vi "Switch Scalar Type.vi"(8 "error in (no error)":errorcluster, 11 "Node Ptr":u64 format="%.0x") -> (0 "error out":errorcluster)   [LabVIEW 2020, in "FPGA Addon System Explorer.lvlib"]
uses:
  FPGA Addon System Explorer.lvlib
  <vilib>/NI VeriStand/Custom Device Tools/Custom Device Utility Library/Search Direction.ctl
  <vilib>/NI VeriStand/Custom Device API/Custom Device Channel.ctl
  <vilib>/NI VeriStand/Custom Device API/Custom Device Channel Type.ctl
  Addon Shared/SubVIs/Constants.vi
  <vilib>/NI VeriStand/Custom Device Tools/Custom Device Utility Library/NI VeriStand - Search for Item by GUID.vi
  <vilib>/NI VeriStand/Custom Device API/Get Item Property (String).vi
  <vilib>/NI VeriStand/Custom Device API/Set Item Property (String).vi
  <vilib>/NI VeriStand/Custom Device API/Custom Device API.lvlib
  Addon Shared/FPGA Addon Shared.lvlib
  <vilib>/NI VeriStand/Custom Device Tools/Custom Device Utility Library/Custom Device Utility Library.lvlib
panel:
  in  "Tag":string
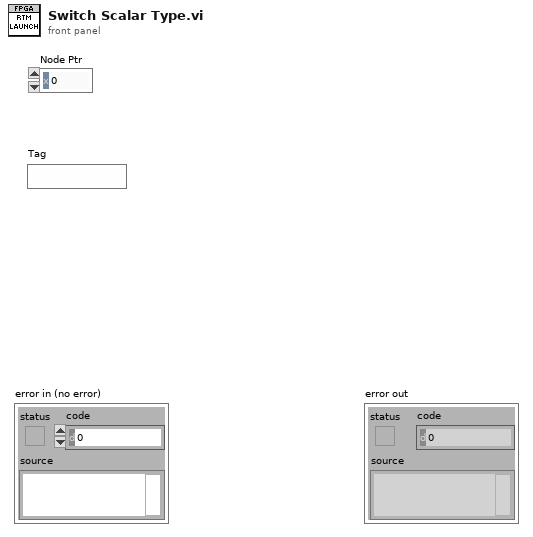
[diagram p1: front panel]
types:
  T1 = typedef "Custom Device Utility Library.lvlib/Search Direction.ctl" = enum16{"Down", "Up"}
  T2 = typedef "Custom Device API.lvlib/Custom Device Item Ref.ctl" = u64
  T3 = typedef "Custom Device API.lvlib/Custom Device Item Info.ctl" = cluster{"Name":string, "Is Channel":bool, "GUID":string, "Is Waveform":bool}
  T4 = typedef "Custom Device API.lvlib/Custom Device Channel.ctl" = cluster{"Type":T5, "Units":string, "Default Value":dbl, "Faultable":bool, "Scalable":bool}
  T5 = typedef "Custom Device API.lvlib/Custom Device Channel Type.ctl" = enum16{"Input", "Output"}
  T6 = enum32{"invalid app kind", "Development System", "Run Time System", "Student Edition", "Embedded LabVIEW", "Evaluation", "Custom"}
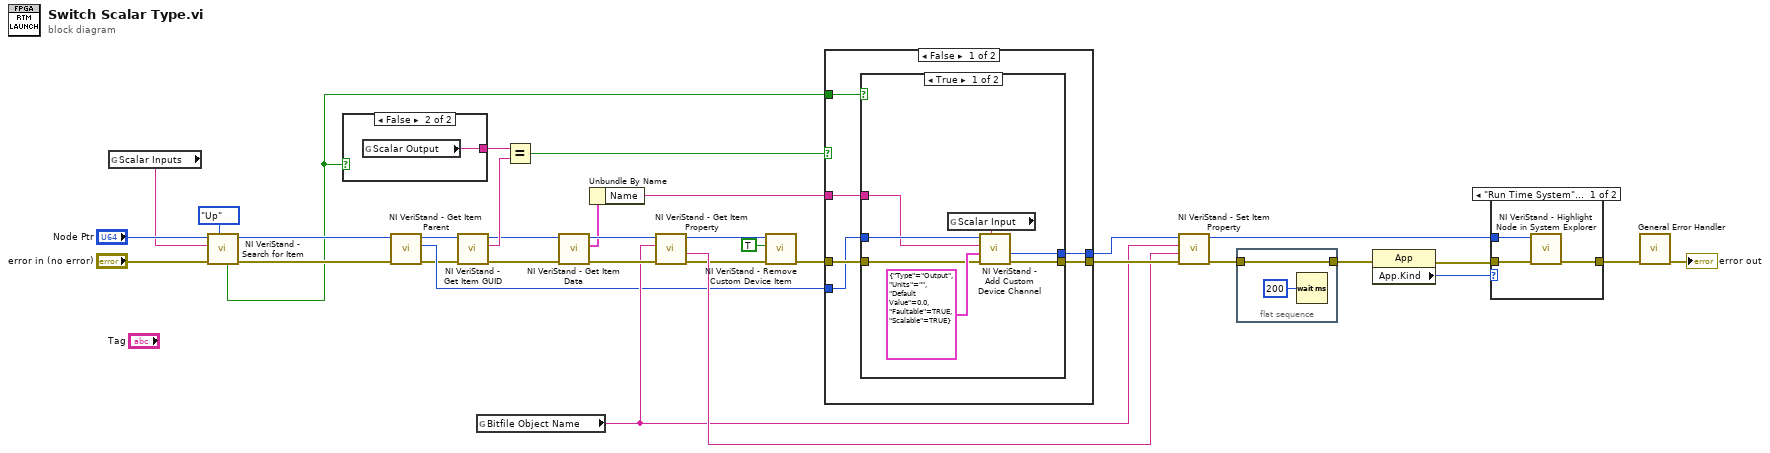
[diagram p0: block diagram]
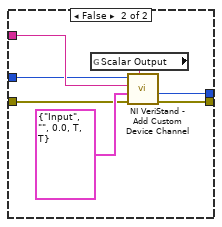
[diagram p3: hidden frame]
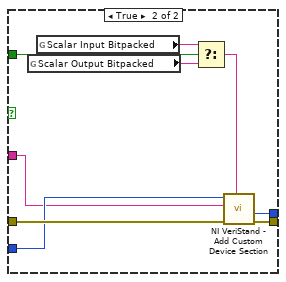
[diagram p4: hidden frame]
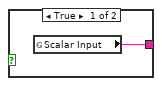
[diagram p5: hidden frame]
diagram:
  n1 = global read "Constants.vi" "Scalar Inputs"() -> (w6:string)
  n2 = call-poly <vilib>:"NI VeriStand - Search for Item.vi"("Direction (Down)"=Search_Direction."Up", "error in"="error in (no error)", "Item GUID"=w6, "Section Ref in"="Node Ptr") -> ("error out"=w8:errorcluster, "Section Ref out"=w7:T2, "Found"=w4:bool)  [unwired: 4 in, 1 out]
  n3 = case shown="False" w4 {
    tunnel: [w35 w36] -> w32
    frame True {
      n4 = global read "Constants.vi" "Scalar Input"() -> (w35:string)
    }
    frame False {
      n5 = global read "Constants.vi" "Scalar Output"() -> (w36:string)
    }
  }
  n6 = call <vilib>:"NI VeriStand - Get Item Parent.vi"("error in (no error)"=w8, "Item Ref in"=w7) -> ("error out"=w11:errorcluster, "Parent Ref"=w12:T2, "Item Ref out"=w31:T2)  [unwired: 6 in, 1 out]
  n7 = call <vilib>:"NI VeriStand - Get Item GUID.vi"("error in (no error)"=w11, "Item Ref in"=w31) -> ("error out"=w20:errorcluster, "GUID"=w34:string, "Item Ref out"=w22:T2)  [unwired: 7 in]
  n8 = global read "Constants.vi" "Bitfile Object Name"() -> (w16:string)
  n9 = Equal?(x=w32, y=w34) -> (x = y?=w28:bool)
  n10 = call <vilib>:"NI VeriStand - Get Item Data.vi"("error in (no error)"=w20, "Item Ref in"=w22) -> ("error out"=w19:errorcluster, "Item Info"=w18:T3, "Item Ref out"=w21:T2)  [unwired: 6 in, 1 out]
  n11 = Unbundle By Name(w18) -> ("Name"=w17:string)
  n12 = call-poly <vilib>:"NI VeriStand - Get Item Property.vi"("error in (no error)"=w19, "Property Name"=w16, "Item Ref in"=w21) -> ("error out"=w24:errorcluster, "Value"=w25:string, "Item Ref out"=w23:T2)  [unwired: 5 in, 1 out]
  n13 = call <vilib>:"NI VeriStand - Remove Custom Device Item.vi"("error in (no error)"=w24, "Force Delete (F)"=TRUE, "Item Ref in"=w23) -> ("error out"=w29:errorcluster)  [unwired: 7 in, 1 out]
  n14 = case shown="False" w28 {
    tunnel: w29 -> [w42 w65]
    tunnel: w12 -> [w38 w64]
    tunnel: w4 -> [w39 w62]
    tunnel: [w41 w60] -> w27
    tunnel: [w40 w59] -> w26
    tunnel: w17 -> [w37 w58]
    frame False {
      n15 = case shown="True" w39 {
        tunnel: w42 -> [w47 w54]
        tunnel: [w46 w53] -> w41
        tunnel: [w45 w52] -> w40
        tunnel: w38 -> [w44 w50]
        tunnel: w37 -> [w43 w51]
        frame True {
          n16 = global read "Constants.vi" "Scalar Input"() -> (w49:string)
          n17 = call <vilib>:"NI VeriStand - Add Custom Device Channel.vi"("GUID (Default Channel)"=w49, "error in (no error)"=w47, "Channel"=T4 {"Type"=enum."Output", "Units"="", "Default Value"=0.0, "Faultable"=TRUE, "Scalable"=TRUE}, "Channel Name"=w43, "Parent Ref in"=w44) -> ("error out"=w46:errorcluster, "Channel Ref"=w45:T2)  [unwired: 3 in, 2 out]
        }
        frame False {
          n18 = global read "Constants.vi" "Scalar Output"() -> (w56:string)
          n19 = call <vilib>:"NI VeriStand - Add Custom Device Channel.vi"("GUID (Default Channel)"=w56, "error in (no error)"=w54, "Channel"=T4 {"Type"=enum."Input", "Units"="", "Default Value"=0.0, "Faultable"=TRUE, "Scalable"=TRUE}, "Channel Name"=w51, "Parent Ref in"=w50) -> ("error out"=w53:errorcluster, "Channel Ref"=w52:T2)  [unwired: 3 in, 2 out]
        }
      }
    }
    frame True {
      n20 = global read "Constants.vi" "Scalar Output Bitpacked"() -> (w61:string)
      n21 = global read "Constants.vi" "Scalar Input Bitpacked"() -> (w63:string)
      n22 = Select(t=w63, s=w62, f=w61) -> (s? t:f=w57:string)
      n23 = call <vilib>:"NI VeriStand - Add Custom Device Section.vi"("GUID (Default Section)"=w57, "error in (no error)"=w65, "Section Name"=w58, "Parent Ref in"=w64) -> ("error out"=w60:errorcluster, "Section Ptr"=w59:T2)  [unwired: 4 in, 2 out]
    }
  }
  n24 = call-poly <vilib>:"NI VeriStand - Set Item Property.vi"("error in (no error)"=w27, "Value"=w25, "Property Name"=w16, "Item Ref in"=w26) -> ("error out"=w13:errorcluster, "Item Ref out"=w14:T2)  [unwired: 5 in, 1 out]
  n25 = flat-sequence {
    tunnel: [w67] -> w3
    tunnel: w13 -> [w67]
    frame #0 {
      n26 = Wait (ms)(milliseconds to wait=u32 200) -> ()  [unwired: 1 out]
    }
  }
  n27 = property class="App"(error in=w3) -> (error out=w1:errorcluster, "App.Kind"=w2:T6)  [unwired: 1 in, 1 out]
  n28 = case shown="\"Run Time System\", Default" w2 {
    tunnel: [w70 w71] -> w15
    tunnel: w14 -> [w69 _]
    tunnel: w1 -> [w68 w71]
    frame "Run Time System", Default {
      n29 = call <vilib>:"NI VeriStand - Highlight Node in System Explorer.vi"("error in (no error)"=w68, "Item Ref in"=w69) -> ("error out"=w70:errorcluster)  [unwired: 8 in, 1 out]
    }
    frame "Development System" {
    }
  }
  n30 = call <vilib>:"General Error Handler.vi"("error in (no error)"=w15) -> ("error out"=→"error out":errorcluster)  [unwired: 10 in, 4 out]
